vi "Set_TriggerOutput_Source.vi"(8 "error in (no error)":errorcluster, 10 "mode":i32(ring) items=["Wavelength", "Time"], 11 ".NET Reference in":refnum<k24>) -> (0 "error out":errorcluster, 3 ".NET Reference out":refnum<k24>)   [LabVIEW 2017]
uses:
  LV_IL_Sample/DLL/InstrumentDLL.dll
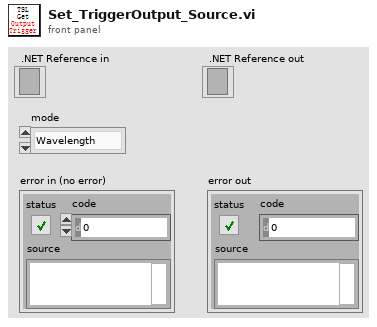
[diagram p1: front panel]
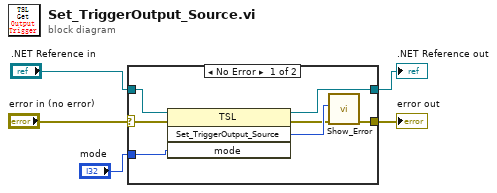
[diagram p0: block diagram]
diagram:
  n1 = case shown="No Error" "error in (no error)" {
    selector: "error in (no error)" -> [w9 w13]
    tunnel: [w6 w13] -> w5
    tunnel: [w12 w14] -> w4
    tunnel: ".NET Reference in" -> [w11 w14]
    tunnel: "mode" -> [w10 _]
    frame No Error {
      n2 = invoke on="调用节点" class="TSL" method="Set_TriggerOutput_Source"(reference=w11, error in=w9, "mode"=w10) -> (reference out=w12:refnum<k24>, error out=w7:errorcluster, "Set_TriggerOutput_Source"=w8:i32)  [unwired: 1 in, 1 out]
      n3 = call "Show_Error.vi"("error in (no error)"=w7, "Error"=w8) -> ("error out"=w6:errorcluster)  [unwired: 9 in]
    }
    frame Error {
    }
  }
  "error out" <- w5
  ".NET Reference out" <- w4
